vi "Check XML for Problems.vi"(8 "error in (no error)":errorcluster, 11 "Node":refnum<k20>) -> (0 "error out":errorcluster, 2 "Has Problems?":bool, 3 "Node out":refnum<k20>)   [LabVIEW 2013]
uses:
  <vilib>/xml/Close Reference(Node).vi
  <vilib>/xml/NI_XML.lvlib
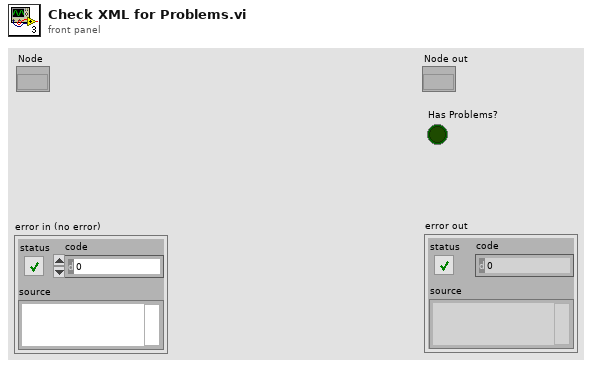
[diagram p1: front panel]
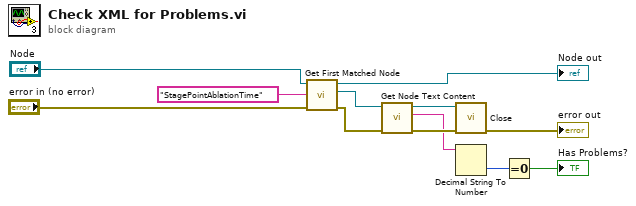
[diagram p0: block diagram]
diagram:
  n1 = call <vilib>:"Get First Matched Node.vi"("error in (no error)"="error in (no error)", "XPath expression"="StagePointAblationTime", "node in"="Node") -> ("error out"=w8:errorcluster, "node result"=w9:refnum<k20>, "node out"=→"Node out":refnum<k20>)  [unwired: 6 in]
  n2 = call <vilib>:"Get Node Text Content.vi"("error in (no error)"=w8, "node in"=w9) -> ("error out"=w10:errorcluster, "node text"=w7:string, "node out"=w11:refnum<k20>)  [unwired: 7 in]
  n3 = call-poly <vilib>:"Close.vi"("error in (no error)"=w10, "node"=w11) -> ("error out"=→"error out":errorcluster)  [unwired: 7 in]
  n4 = Decimal String To Number(string=w7) -> (number=w6:i32)  [unwired: 2 in, 1 out]
  n5 = Equal To 0?(x=w6) -> (x = 0?=→"Has Problems?":bool)
